vi "ExSimple.vi"() -> ()   [LabVIEW 2010]
panel:
  in  "stop":bool
  in  "Detecotr (only available for NCL)":u32=1 min=1 max=3 step=1
  in  "Num of Reads to average":u32=1 min=1 step=1
  in  "Gain Range":u32 max=4 step=1
  in  "Integraion / Exposure ms":dbl=1.0 min=1.0 step=1.0 format="%.2f"
  in  "Detector Type":u32=1 min=1 max=3 step=1
  in  "Bi Polar Enable":bool
  in  "High Volts":dbl format="%.2f"
  in  "High Volts Enable":bool
  out "Detector Type":u32
  out "Bi Polar":bool
  out "Gain Value":dbl format="%.2f"
  out "Gain Range":dbl format="%.2f"
  out "Integraion time ms":dbl format="%.2f"
  out "HV Status":bool
  out "HV Volts":dbl format="%.2f"
  out "Get Ave Rds":u32
  out "reserve 2":u32
  out "reserve 1":u32
  out "Voltage":dbl format="%.2f"
  out "error out":errorcluster
  in  "error in (no error)":errorcluster
  # "1 :  Current\n 2 :  Voltage\n 3 :  Photon Counting"
  # "Minimum is 1.0 ms\nPractical minimum 10.0 ms\nTypical 100.0 ms\nmaximum is 65 sec (65535ms)"
  # "0 : 1x\n1 :  2x\n2 :  4x\n3 : 50x\n4 : 200x"
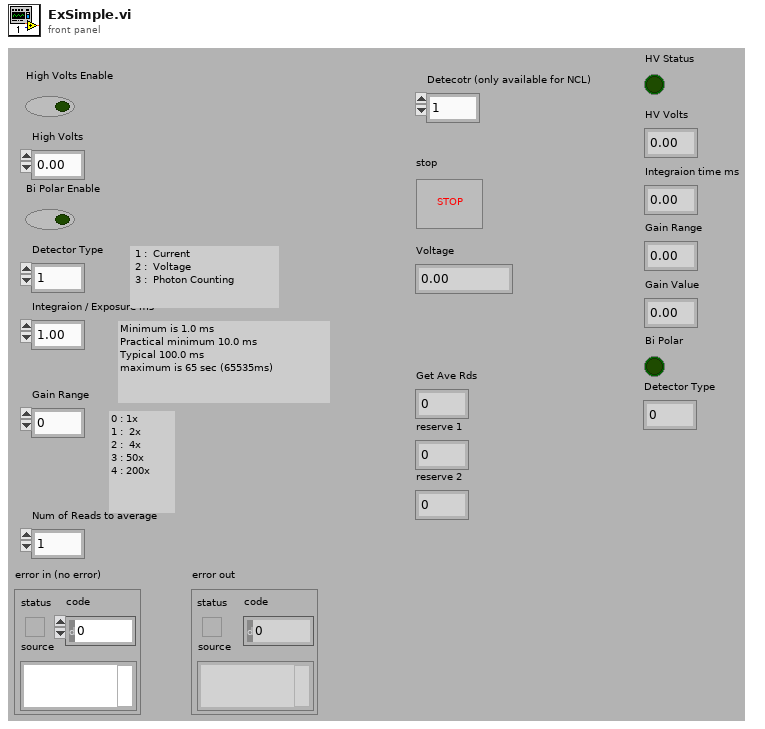
[diagram p1: front panel]
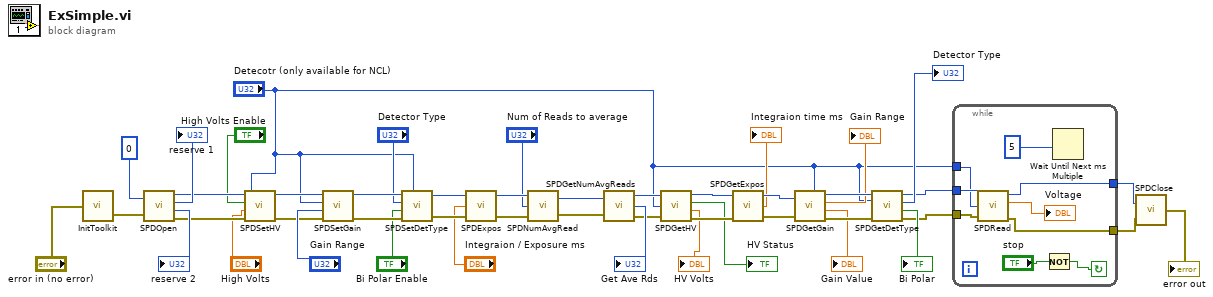
[diagram p0: block diagram]
diagram:
  n1 = call <userlib>:"InitToolkit.vi"("error in"="error in (no error)") -> ("error out"=w45:errorcluster)
  n2 = call <userlib>:"SPDOpen.vi"("Device ID"=0, "error in (no error)"=w45) -> ("SPD Handle"=w24:u32, "reserved 1"=→"reserve 1":u32, "reserved 2"=→"reserve 2":u32, "error out"=w25:errorcluster)
  n3 = call <userlib>:"SPDSetHV.vi"("SPD Handle"=w24, "HV enable/disable"="High Volts Enable", "Volts"="High Volts", "error in (no error)"=w25, "SPD Number"="Detecotr (only available for NCL)") -> ("SPD Handle"=w19:u32, "error out"=w20:errorcluster)
  n4 = call <userlib>:"SPDSetGain.vi"("error in (no error)"=w20, "Gain Range"="Gain Range", "Detector Number"="Detecotr (only available for NCL)", "SPD Handle"=w19) -> ("error out"=w18:errorcluster, "SPD Handle"=w17:u32)
  n5 = call <userlib>:"SPDSetDetType.vi"("SPD Handle"=w17, "Detector Type"="Detector Type", "BiPolar switch"="Bi Polar Enable", "error in (no error)"=w18, "SPD Number"="Detecotr (only available for NCL)") -> ("SPD Handle"=w13:u32, "error out"=w14:errorcluster)
  n6 = call <userlib>:"SPDExpos.vi"("error in (no error)"=w14, "Integration Time (ms)"="Integraion / Exposure ms", "SPD Handle"=w13) -> ("error out"=w11:errorcluster, "SPD Handle"=w10:u32)
  n7 = call <userlib>:"SPDNumAvgRead.vi"("error in (no error)"=w11, "Number to average Reads"="Num of Reads to average", "SPD Handle"=w10) -> ("error out"=w9:errorcluster, "SPD Handle"=w8:u32)
  n8 = call <userlib>:"SPDGetNumAvgReads.vi"("SPD Handle"=w8, "error in (no error)"=w9) -> ("SPD Handle"=w26:u32, "Number of Averages"=→"Get Ave Rds":u32, "error out"=w27:errorcluster)
  n9 = call <userlib>:"SPDGetHV.vi"("SPD Handle"=w26, "Detector Number"="Detecotr (only available for NCL)", "error in (no error)"=w27) -> ("SPD Handle"=w37:u32, "HV Status (ON/OFF)"=→"HV Status":bool, "HV Volts"=→"HV Volts":dbl, "error out"=w40:errorcluster)
  n10 = call <userlib>:"SPDGetExpos.vi"("error in (no error)"=w40, "SPD Handle"=w37) -> ("error out"=w39:errorcluster, "Integration time in ms"=→"Integraion time ms":dbl, "SPD Handle"=w36:u32)  [unwired: 1 in]
  n11 = call <userlib>:"SPDGetGain.vi"("Detector Number"="Detecotr (only available for NCL)", "error in (no error)"=w39, "SPD Handle"=w36) -> ("error out"=w38:errorcluster, "Gain value"=→"Gain Value":dbl, "Gain Range"=→"Gain Range":dbl, "SPD Handle"=w35:u32)
  n12 = call <userlib>:"SPDGetDetType.vi"("SPD Handle"=w35, "SPD Number"="Detecotr (only available for NCL)", "error in (no error)"=w38) -> ("SPD Handle"=w5:u32, "Detector Type"=→"Detector Type":u32, "BiPolar state"=→"Bi Polar":bool, "error out"=w6:errorcluster)
  n13 = while {
    tunnel: w6 -> [w55]
    tunnel: w5 -> [w54]
    tunnel: "Detecotr (only available for NCL)" -> [w53]
    tunnel: [w51] -> w3
    tunnel: [w50] -> w2
    stop <- w48 continue-if-true
    n14 = call <userlib>:"SPDRead.vi"("SPD Handle"=w54, "Detector Number"=w53, "error in (no error)"=w55) -> ("SPD Handle"=w51:u32, "SPD Value"=→"Voltage":dbl, "error out"=w50:errorcluster)  [unwired: 1 out]
    n15 = Not(x="stop") -> (.not. x?=w48:bool)
    n16 = Wait Until Next ms Multiple(millisecond multiple=5) -> ()  [unwired: 1 out]
  }
  n17 = call <userlib>:"SPDClose.vi"("error in (no error)"=w2, "SPD Handle"=w3) -> ("error out"=→"error out":errorcluster)
